vi "vxi11.vi"() -> ()   [LabVIEW 2011]
panel:
  out "error out":errorcluster
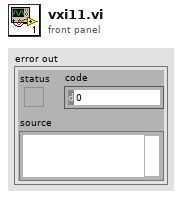
[diagram p1: front panel]
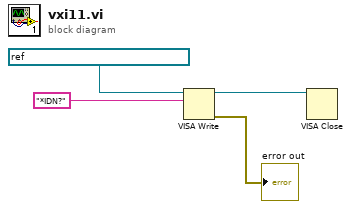
[diagram p0: block diagram]
diagram:
  n1 = VISA Write(VISA resource name=refnum<visa-resource-name> "TCPIP::192.168.56.102::INSTR", write buffer="*IDN?") -> (VISA resource name out=w1:refnum<visa-resource-name>, error out=→"error out":errorcluster)  [unwired: 1 in, 1 out]
  n2 = VISA Close(VISA resource name=w1) -> ()  [unwired: 1 in, 1 out]
